vi "Exemple_Metrics_Roc_Curve.vi"() -> ()   [LabVIEW 2020]
uses:
  Objet/3 - Model selection and evaluation/3.3 - Metrics and scoring/roc_curve/Roc_Curve.vi
panel:
  out "Data":T1
  out "error out":errorcluster caption="sortie d'erreur"
  in  "roc_curve":T2={"pos_label"={"dtype_pos_label"="int", "pos_label"="2"}, "sample_weight"=[], "drop_intermediate"=TRUE, "Returns"="fpr"}
  in  "error in (no error)":errorcluster caption="entrée d'erreur (pas d'erreur)"
  in  "y_score":string[][](array[string])=[["0,1"], ["0,4"], ["0,35"], ["0,8"]]
  in  "y_true":string[][](array[string])=[["1"], ["1"], ["2"], ["2"]]
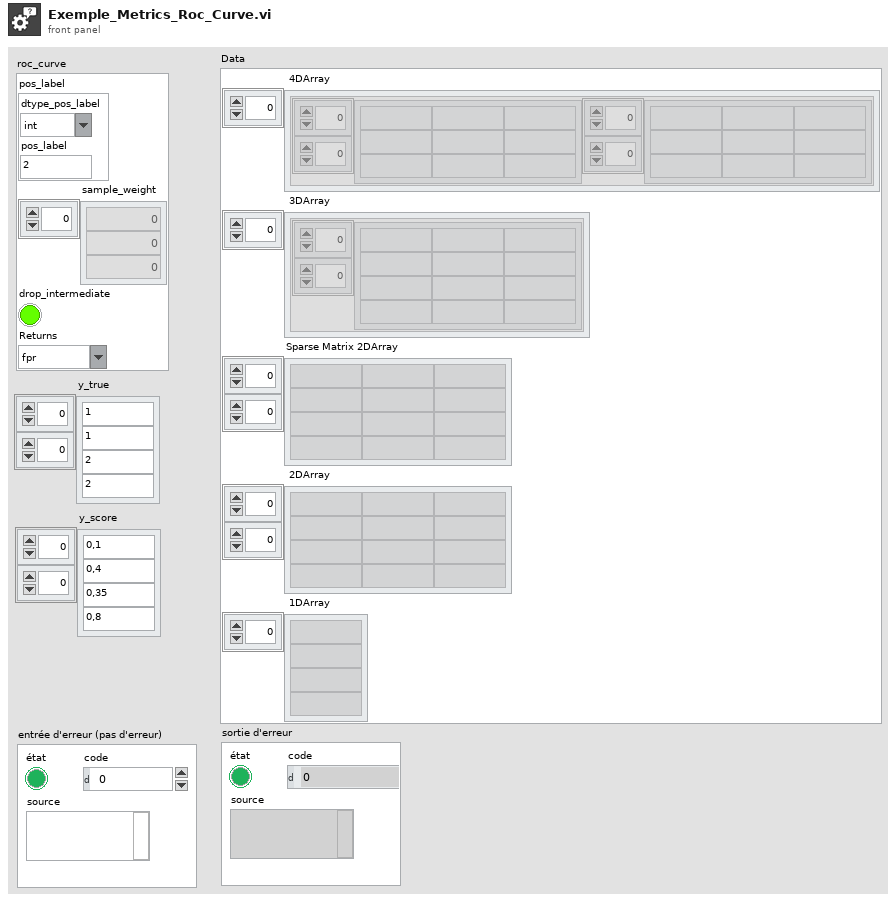
[diagram p1: front panel]
types:
  T1 = cluster{" 4DArray":cluster{"1":string[][], "2":string[][]}[], " 3DArray":cluster{"Tableau":string[][]}[], "Sparse Matrix 2DArray":string[][], " 2DArray":string[][], " 1DArray":string[]}
  T2 = cluster{"pos_label":cluster{"dtype_pos_label":string, "pos_label":string}, "sample_weight":dbl[], "drop_intermediate":bool, "Returns":string}
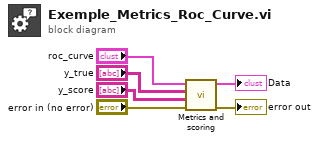
[diagram p0: block diagram]
diagram:
  n1 = call-poly "Metrics and scoring.vi"("error in (no error)"="error in (no error)", "y_score"="y_score", "y_true"="y_true", "roc_curve"="roc_curve") -> ("error out"=→"error out":errorcluster, "Data"=→"Data":T1)  [unwired: 6 in]
